vi "Write Cell Laser Diode Signal.vi"(8 "error in":errorcluster, 10 "lasDiodeData":waveform(i16), 11 "PAS Data in":refnum<class "PAS Data.lvclass">) -> (0 "error out":errorcluster, 3 "PAS Data out":refnum<class "PAS Data.lvclass">)   [LabVIEW 2015, in "PAS Library.lvlib" / "PAS Data.lvclass"]
uses:
  PAS Data.lvclass
  PAS Data.lvclass/PAS Data.ctl
  Cell/PAS Cell Data.lvclass
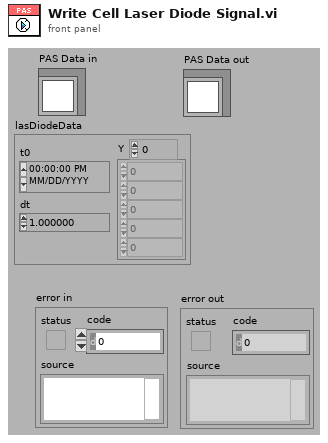
[diagram p1: front panel]
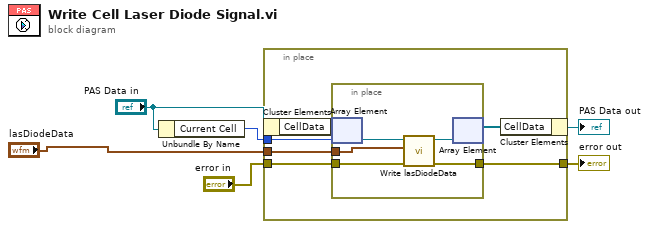
[diagram p0: block diagram]
diagram:
  n1 = Unbundle By Name("PAS Data in") -> ("Current Cell"=w2:i32)
  n2 = in-place {
    in-place-border: w2 -> [w12]
    in-place-border: "error in" -> [w11]
    in-place-border: [w10] -> w5
    in-place-border: "lasDiodeData" -> [w7]
    n3 = in-place-cluster #1("PAS Data in") -> ("CellData"=w9:refnum<class "PAS Cell Data.lvclass">[])
    n4 = in-place {
      in-place-border: w11 -> [w16]
      in-place-border: [w14] -> w10
      in-place-border: w7 -> [w13]
      n5 = in-place-array #2(w9, w12) -> (w17:refnum<class "PAS Cell Data.lvclass">)
      n6 = call "Write lasDiodeData.vi"("error in"=w16, "lasDiodeData"=w13, "PAS Cell Data in"=w17) -> ("error out"=w14:errorcluster, "PAS Cell Data out"=w15:refnum<class "PAS Cell Data.lvclass">)  [unwired: 7 in]
      n7 = in-place-array #2(w15) -> (w8:refnum<class "PAS Cell Data.lvclass">[])  [unwired: 1 out]
    }
    n8 = in-place-cluster #1("CellData"=w8) -> (→"PAS Data out":refnum<class "PAS Data.lvclass">)
  }
  "error out" <- w5
